vi "Calibration Routine State Machine.vi"(8 "error in (no error)":errorcluster, 11 "Calibration Array in":T1[](array[typedef])) -> (0 "error out":errorcluster, 3 "Calibration Array out":T1[](array[typedef]))   [LabVIEW 2020, in "Acquisition.lvlib"]
doc: "_____\nBased on DQMH Project Template 6.0.0.91."
uses:
  Acquisition.lvlib
  CML Shared/Calibration Values--cluster.ctl
  Calibration Routine State--enum.ctl
  CML Shared/CML Shared.lvlib
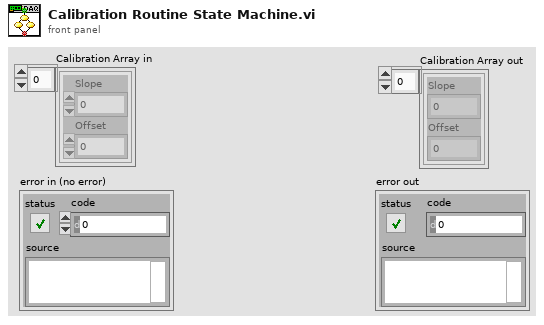
[diagram p1: front panel]
types:
  T1 = typedef "CML Shared.lvlib/Calibration Values--cluster.ctl" = cluster{"Slope":dbl, "Offset":dbl}
  T2 = typedef "Acquisition.lvlib/Calibration Routine State--enum.ctl" = enum16{"Start", "Start External Cal Source", "Measure Source", "Stop External Cal Source", "Calculate Calibration Fit", "Done"}
  T3 = typedef "Acquisition.lvlib/Request Events--cluster.ctl" = cluster{"Stop Module":refnum<user-event>, "Show Panel":refnum<user-event>, "Hide Panel":refnum<user-event>, "Get Module Execution Status":refnum<user-event>, "Show Diagram":refnum<user-event>, "Stop Acquiring":refnum<user-event>, "Wakeup Helper Loop":refnum<user-event>, "Change Settings":refnum<user-event>, "Calibrate DAQ":refnum<user-event>, "Start Acquiring":refnum<user-event>}
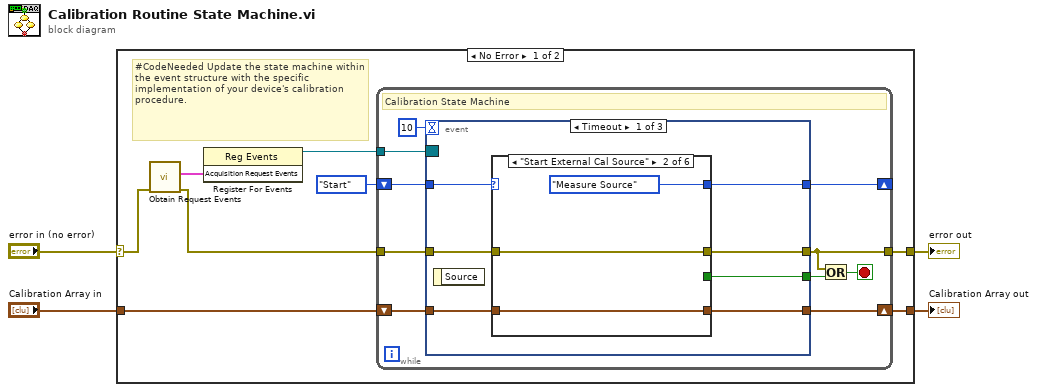
[diagram p0: block diagram]
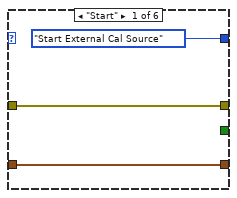
[diagram p2: hidden frame]
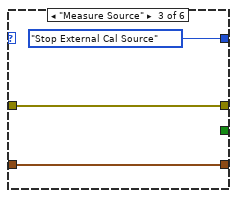
[diagram p3: hidden frame]
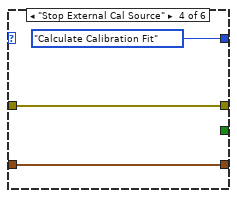
[diagram p4: hidden frame]
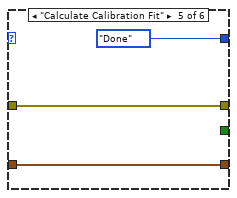
[diagram p5: hidden frame]
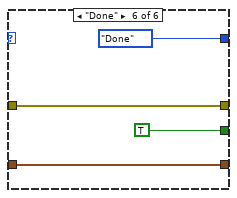
[diagram p6: hidden frame]
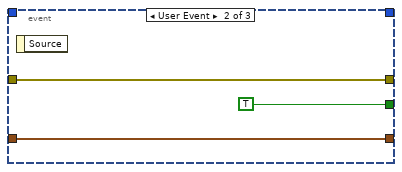
[diagram p7: hidden frame]
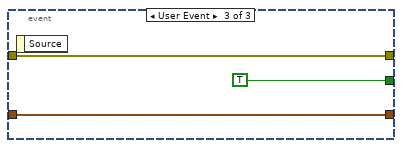
[diagram p8: hidden frame]
diagram:
  n1 = case shown="No Error" "error in (no error)" {
    selector: "error in (no error)" -> [w12 w56]
    tunnel: [w7 w56] -> w4
    tunnel: "Calibration Array in" -> [w6 w55]
    tunnel: [w5 w55] -> w1
    frame No Error {
      # "#CodeNeeded Update the state machine within the event structure with the specific implementation of your device's calibration procedure."
      n2 = call "Obtain Request Events.vi"("error in (no error)"=w12) -> ("error out"=w8:errorcluster, "Acquisition Request Events"=w10:T3)  [unwired: 9 in]
      n3 = register-events(w10) -> (reference out=w9:refnum<event-registration>)  [unwired: 2 in, 1 out]
      n4 = while {
        shift-right: [w21] -> _
        shift-left: Calibration_Routine_State--enum."Start" -> [w22]
        tunnel: w9 -> [w20]
        shift-right: [w15] -> w5
        shift-left: w6 -> [w16]
        tunnel: w8 -> [w18]
        tunnel: [w14] -> w7
        stop <- w17 stop-if-true
        # "Calibration State Machine"
        n5 = event shown="[0] Timeout" {
          selector: w20 -> [_ _ _]
          dyn-events: _ -> [_ _ _]
          timeout: 10 -> [_ _ _]
          tunnel: w22 -> [w29 _ _]
          tunnel: [w28 _ _] -> w21
          tunnel: [w27 TRUE TRUE] -> w13
          tunnel: w18 -> [w26 w49 w52]
          tunnel: [w25 w49 w52] -> w14
          tunnel: w16 -> [w23 w50 w53]
          tunnel: [w24 w50 w53] -> w15
          event Timeout {
            n6 = event-data() -> ()  [unwired: 1 in, 1 out]
            n7 = case shown="\"Start External Cal Source\"" w29 {
              tunnel: [Calibration_Routine_State--enum."Start External Cal Source" Calibration_Routine_State--enum."Measure Source" Calibration_Routine_State--enum."Stop External Cal Source" Calibration_Routine_State--enum."Calculate Calibration Fit" Calibration_Routine_State--enum."Done" Calibration_Routine_State--enum."Done"] -> w28
              tunnel: [_ _ _ _ _ TRUE] -> w27
              tunnel: w26 -> [w31 w34 w37 w40 w43 w46]
              tunnel: [w31 w34 w37 w40 w43 w46] -> w25
              tunnel: [w30 w33 w36 w39 w42 w45] -> w24
              tunnel: w23 -> [w30 w33 w36 w39 w42 w45]
              frame "Start" {
              }
              frame "Start External Cal Source" {
              }
              frame "Measure Source" {
              }
              frame "Stop External Cal Source" {
              }
              frame "Calculate Calibration Fit" {
              }
              frame "Done" {
              }
            }
          }
          event User Event {
            n8 = event-data() -> ()  [unwired: 1 in, 1 out]
          }
          event User Event {
            n9 = event-data() -> ()  [unwired: 1 in, 1 out]
          }
        }
        n10 = Or(x=w14, y=w13) -> (x .or. y?=w17:bool)
      }
    }
    frame Error {
    }
  }
  "error out" <- w4
  "Calibration Array out" <- w1
